vi "CreateProduct.vi"(8 "error in (no error)":errorcluster, 11 "Creator":refnum<class "Creator.lvclass">) -> (0 "error out":errorcluster, 2 "Product":refnum<class "Product.lvclass">, 3 "Creator":refnum<class "Creator.lvclass">)   [LabVIEW 2020, in "FactoryMethod.lvlib" / "FactoryMethodLazyEvaluation.lvlib" / "Creator.lvclass"]
uses:
  Creator.lvclass
  Product/Product.lvclass
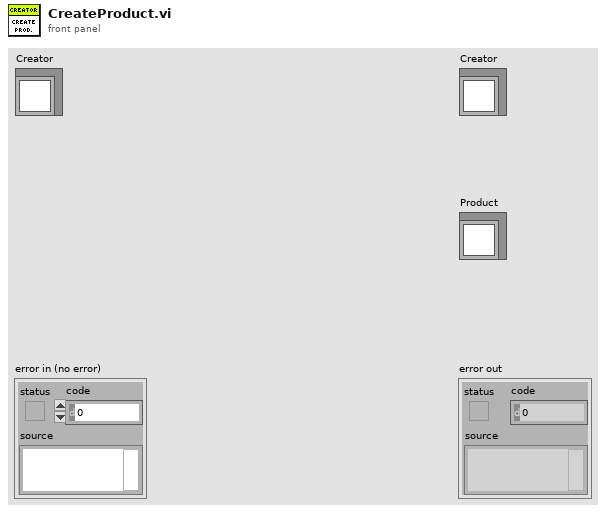
[diagram p1: front panel]
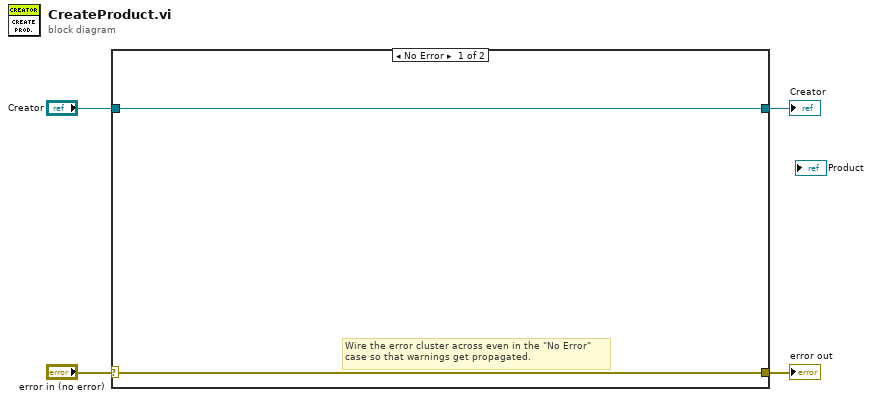
[diagram p0: block diagram]
diagram:
  n1 = case shown="No Error" "error in (no error)" {
    selector: "error in (no error)" -> [w5 w8]
    tunnel: [w5 w8] -> w3
    tunnel: [w6 w7] -> w2
    tunnel: "Creator" -> [w6 w7]
    frame No Error {
      # "Wire the error cluster across even in the \"No Error\"\ncase so that warnings get propagated."
    }
    frame Error {
    }
  }
  "error out" <- w3
  "Creator" <- w2
